vi "PortSet.vi"(8 "error in (no error)":errorcluster caption="错误输入（无错误）") -> (0 "error out":errorcluster caption="错误输出", 1 "PC端-协议类型 2":enum16{"TCP服务器Server", "TCP客户端Client"}(ring), 2 "通信端口:":dbl, 3 "CANET地址格式如：192.168.0.178":string)   [LabVIEW 2013]
panel:
  in  "PC端-协议类型":enum16{"TCP服务器Server", "TCP客户端Client"}(ring)
  in  "确定按钮":bool
  in  "CANET-IP地址：格式如：192.168.0.178\nPC端作为客户端使用时需要填写":string
  in  "通信端口":u32
  # "波特率需要使用专用\n工具进行设置"
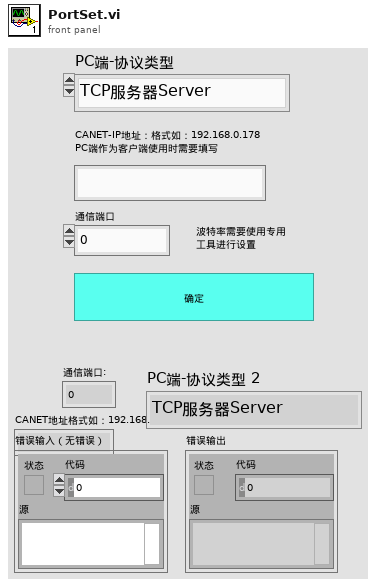
[diagram p1: front panel]
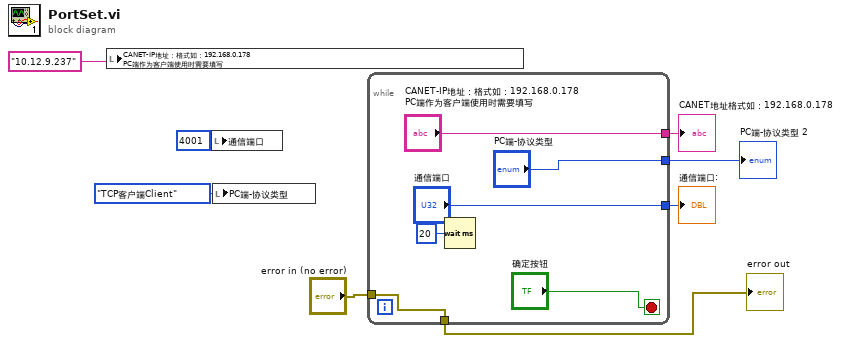
[diagram p0: block diagram]
diagram:
  n1 = local write "CANET-IP地址：格式如：192.168.0.178\nPC端作为客户端使用时需要填写"("10.12.9.237" ("CANET地址：格式如：192.168.0.178")) -> ()
  n2 = local write "通信端口"(u32 4001 ("通信端口")) -> ()
  n3 = local write "PC端-协议类型"(enum16{"TCP服务器Server", "TCP客户端Client"}."TCP客户端Client" ("PC端-协议类型")) -> ()
  n4 = while {
    tunnel: ["CANET-IP地址：格式如：192.168.0.178\nPC端作为客户端使用时需要填写"] -> w8
    tunnel: ["通信端口"] -> w7
    tunnel: "error in (no error)" -> [w10]
    tunnel: [w10] -> w5
    tunnel: ["PC端-协议类型"] -> w2
    stop <- "确定按钮" stop-if-true
    n5 = Wait (ms)(milliseconds to wait=u32 20 ("等待时间（毫秒）")) -> ()  [unwired: 1 out]
  }
  "CANET地址格式如：192.168.0.178" <- w8
  "通信端口:" <- w7
  "error out" <- w5
  "PC端-协议类型 2" <- w2
